vi "Read Attributes Metadata.vi"(11 "Attributes in":refnum<class "Attributes.lvclass">) -> (2 "Attributes Metadata":refnum<class "Attributes Metadata.lvclass">)   [LabVIEW 2020, in "jettl.lvlib" / "Attributes.lvclass"]
uses:
  Attributes.lvclass
  Attributes Metadata/Attributes Metadata.lvclass
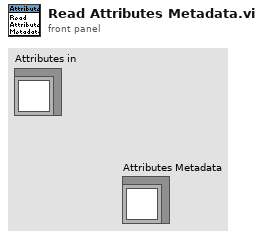
[diagram p1: front panel]
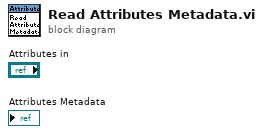
[diagram p0: block diagram]
diagram:
